vi "Text-Format Bytes.vi"(7 "Bytes":i64, 13 "Precision":i32=2) -> (8 "resulting string":string)   [LabVIEW 2020]
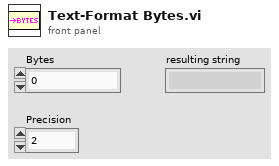
[diagram p1: front panel]
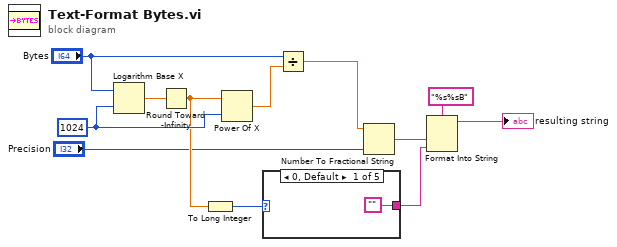
[diagram p0: block diagram]
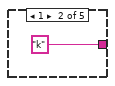
[diagram p2: hidden frame]
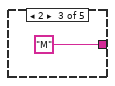
[diagram p3: hidden frame]
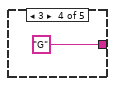
[diagram p4: hidden frame]
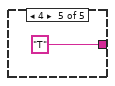
[diagram p5: hidden frame]
diagram:
  w11 = i64 1024 ("x")
  n1 = Logarithm Base X(1:w11, 2:"Bytes") -> (0:w12:dbl)
  n2 = Round Toward -Infinity(1:w12) -> (0:w8:dbl)
  n3 = To Long Integer(number=w8) -> (32bit integer=w7:i32)
  n4 = Power Of X(1:w11, 2:w8) -> (0:w9:dbl)
  n5 = case shown="0, Default" w7 {
    tunnel: ["" "k" "M" "G" "T"] -> w5
    frame 0, Default {
    }
    frame 1 {
    }
    frame 2 {
    }
    frame 3 {
    }
    frame 4 {
    }
  }
  n6 = Divide(x="Bytes", y=w9) -> (x/y=w3:dbl)
  n7 = Number To Fractional String(number=w3, precision (6)="Precision") -> (F-format string=w2:string)  [unwired: 2 in]
  n8 = Format Into String(format string="%s%sB", w2, w5) -> (resulting string=→"resulting string":string)  [unwired: 2 in, 1 out]
